vi "Large int-multiplty a by 0 to 10.vi"(8 "error in (no error)":errorcluster, 10 "b (0 to 10 inclusive)":u32, 11 "a = Large int (decimal)":string) -> (0 "error out":errorcluster, 2 "T = \"a\" is an integer":bool, 3 "c = a x b":string)   [LabVIEW 2021, in "Numeric Utilities.lvlib"]
uses:
  Numeric Utilities.lvlib
panel:
  out "Loop iteration":i32
  # "Development\ncontrols/indicators useful for development and testing, but which are not outputs of the VI"
  # "Input\nInputs to the VI"
  # "Output\nOutputs of the VI"
  # "Description\n\nBlank VI with error handling case. \n\nSummarize the use of this VI in this space."
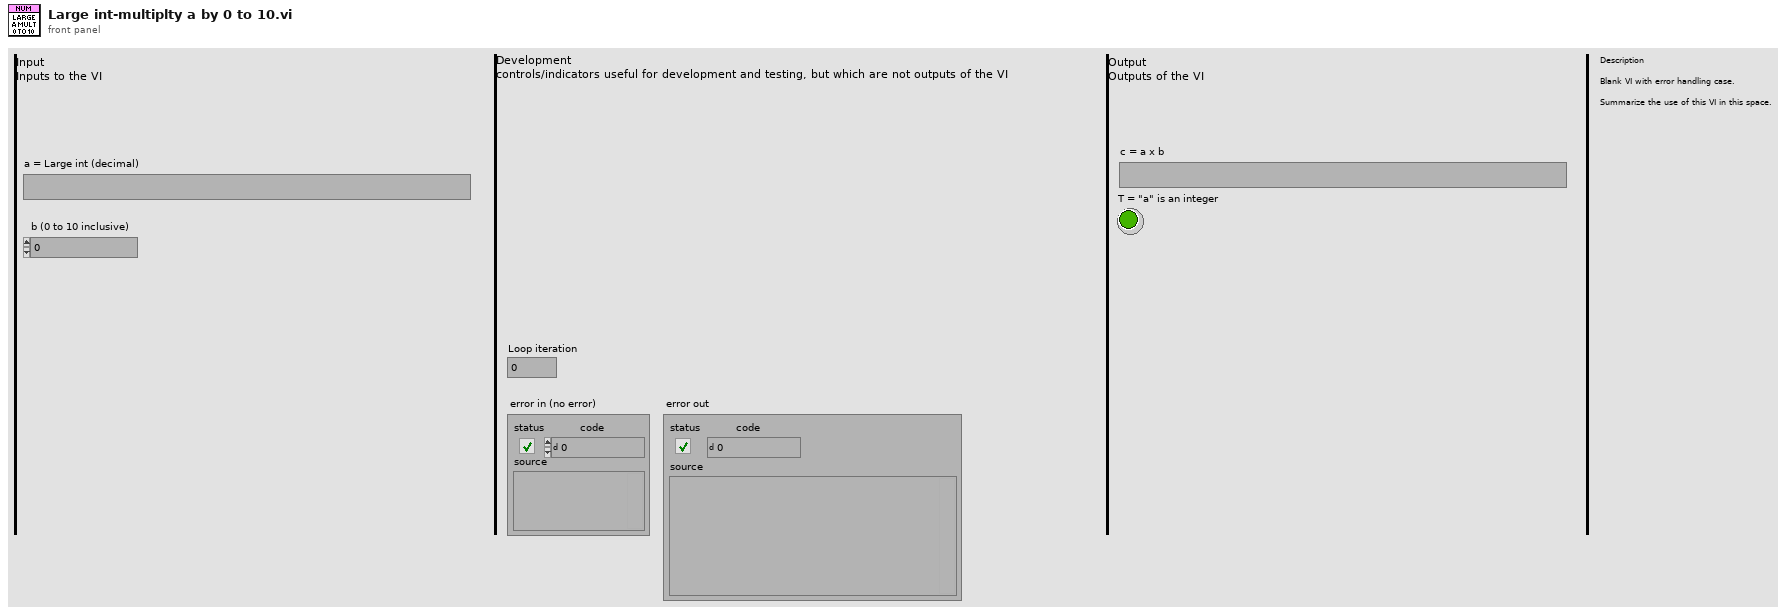
[diagram p1: front panel]
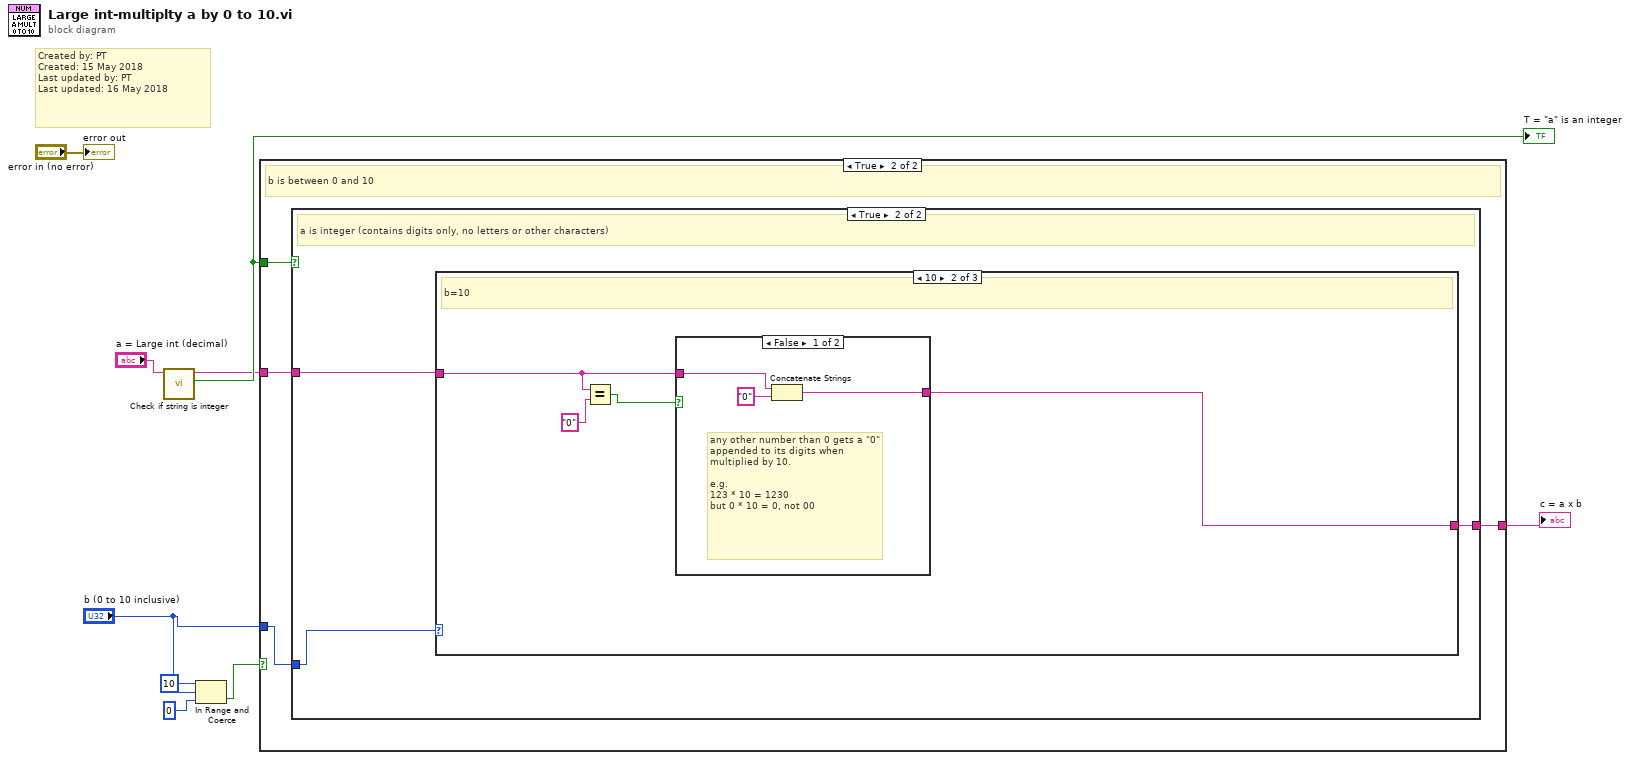
[diagram p0: block diagram]
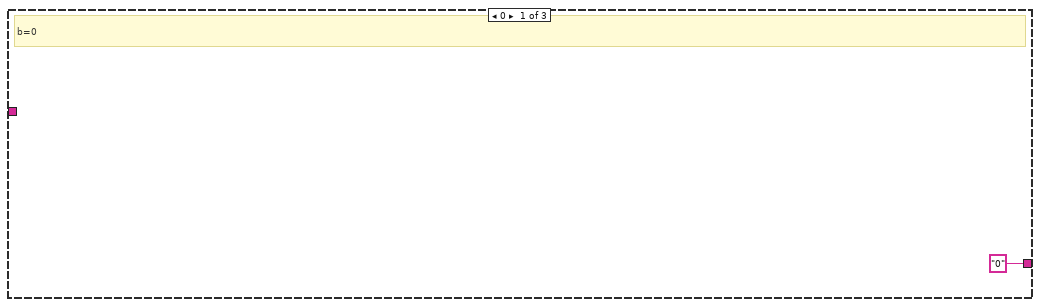
[diagram p4: hidden frame]
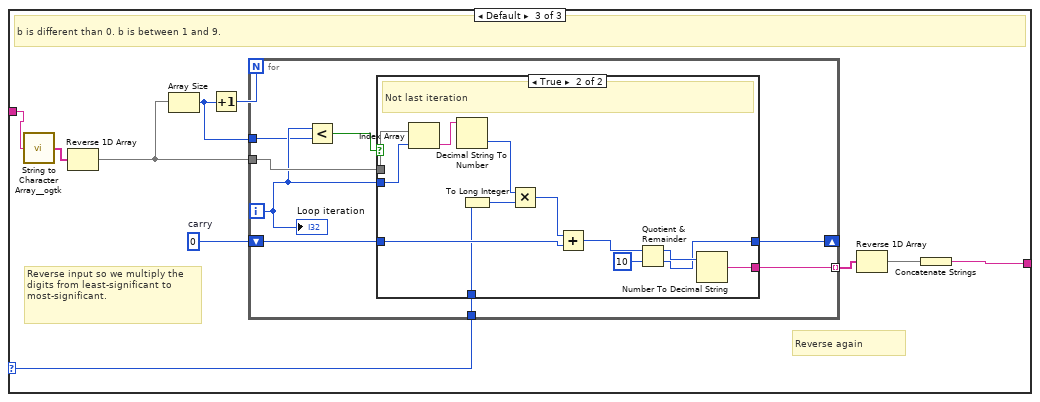
[diagram p6: hidden frame]
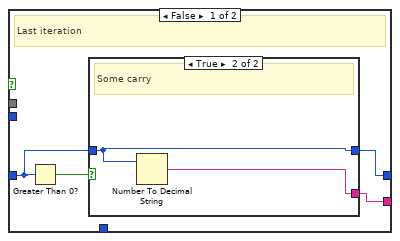
[diagram p7: hidden frame]
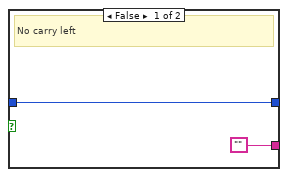
[diagram p8: hidden frame]
diagram:
  # "Created by: PT\nCreated: 15 May 2018\nLast updated by: PT\nLast updated: 16 May 2018"
  n1 = call "Check if string is integer.vi"("string in"="a = Large int (decimal)") -> ("T = string contains an integer"=w2:bool, "string out (duplicate)"=w1:string)  [unwired: 8 in, 1 out]
  "T = \"a\" is an integer" <- w2
  n2 = In Range and Coerce(upper limit=u32 10, x="b (0 to 10 inclusive)", lower limit=u32 0) -> (In Range?=w5:bool)  [unwired: 1 out]
  n3 = case shown="True" w5 {
    tunnel: [_ w13] -> w9
    tunnel: "b (0 to 10 inclusive)" -> [_ w12]
    tunnel: w2 -> [_ w11]
    tunnel: w1 -> [_ w10]
    frame False {
      # "b is not between 0 and 10"
    }
    frame True {
      # "b is between 0 and 10"
      n4 = case shown="True" w11 {
        tunnel: [_ w16] -> w13
        tunnel: w12 -> [_ w15]
        tunnel: w10 -> [_ w14]
        frame False {
          # "Input is not an integer"
        }
        frame True {
          # "a is integer (contains digits only, no letters or other characters)"
          n5 = case shown="10" w15 {
            selector: w15 -> [_ _ w29]
            tunnel: ["0" w21 w33] -> w16
            tunnel: w14 -> [_ w20 w26]
            frame 0 {
              # "b=0"
            }
            frame 10 {
              # "b=10"
              n6 = Equal?(x=w20, y="0" ("string")) -> (x = y?=w18:bool)
              n7 = case shown="False" w18 {
                tunnel: w20 -> [w24 w25]
                tunnel: [w22 w25] -> w21
                frame False {
                  # "any other number than 0 gets a \"0\" appended to its digits when multiplied by 10.\n\ne.g.\n123 * 10 = 1230\nbut 0 * 10 = 0, not 00"
                  n8 = Concatenate Strings(w24, "0" ("string")) -> (w22:string)
                }
                frame True {
                  # "0 x 10 = 0"
                }
              }
            }
            frame Default {
              w35 = 0  # carry
              # "Reverse input so we multiply the digits from least-significant to most-significant."
              # "Reverse again"
              # "b is different than 0. b is between 1 and 9."
              n9 = call <userlib>:"String to Character Array__ogtk.vi"("Input String"=w26) -> ("Character Array"=w27:string[])
              n10 = Reverse 1D Array(array=w27) -> (reversed array=w28:string[])
              n11 = Array Size(array=w28) -> (size(s)=w30:i32)
              n12 = Increment(x=w30) -> (x+1=w31:i32)
              n13 = for {
                N: w31 -> [_]
                tunnel: w28 -> [w43]
                shift-right: [w40] -> _
                shift-left: w35 -> [w42]
                tunnel: [w41] -> w34 mode=indexing
                tunnel: w30 -> [w38]
                tunnel: w29 -> [w36]
                i -> [w39]
                n14 = Less?(x=w39, y=w38) -> (x < y?=w37:bool)
                n15 = case shown="True" w37 {
                  tunnel: w43 -> [_ w64]
                  tunnel: w42 -> [w44 w61]
                  tunnel: [w46 w58] -> w41
                  tunnel: [w45 w55] -> w40
                  tunnel: w39 -> [_ w53]
                  tunnel: w36 -> [_ w52]
                  frame False {
                    # "Last iteration"
                    n16 = Greater Than 0?(x=w44) -> (x > 0?=w47:bool)
                    n17 = case shown="True" w47 {
                      tunnel: ["" w51] -> w46
                      tunnel: [w48 w50] -> w45
                      tunnel: w44 -> [w48 w50]
                      frame False {
                        # "No carry left"
                      }
                      frame True {
                        # "Some carry"
                        n18 = Number To Decimal String(number=w50) -> (decimal integer string=w51:string)  [unwired: 1 in]
                      }
                    }
                  }
                  frame True {
                    # "Not last iteration"
                    n19 = Index Array(array=w64, index=w53) -> (element=w54:string)
                    n20 = Decimal String To Number(string=w54) -> (number=w63:i32)  [unwired: 2 in, 1 out]
                    n21 = To Long Integer(number=w52) -> (32bit integer=w62:i32)
                    n22 = Multiply(x=w63, y=w62) -> (x*y=w57:i32)
                    n23 = Add(x=w57, y=w61) -> (x+y=w60:i32)
                    n24 = Quotient & Remainder(x=w60, y=10) -> (x-y*floor(x/y)=w56:i32, floor(x/y)=w55:i32)
                    n25 = Number To Decimal String(number=w56) -> (decimal integer string=w58:string)  [unwired: 1 in]
                  }
                }
                "Loop iteration" <- w39
              }
              n26 = Reverse 1D Array(array=w34) -> (reversed array=w32:string[])
              n27 = Concatenate Strings(w32) -> (w33:string)
            }
          }
        }
      }
    }
  }
  "c = a x b" <- w9
  "error out" <- "error in (no error)"
